vi "Test Formula.vi"() -> ()   [LabVIEW 2021]
uses:
  WHH Formula Data.ctl
panel:
  in  "alpha_Maki":dbl
  out "Array - Numeric":dbl[](array[numeric])
  out "XY Graph":cluster{dbl[], "Steps":dbl[]}(graph)
  in  "Number of steps":i32=20
  in  "End":dbl=0.99
  in  "Start":dbl=1e-05
  in  "t":dbl=0.5
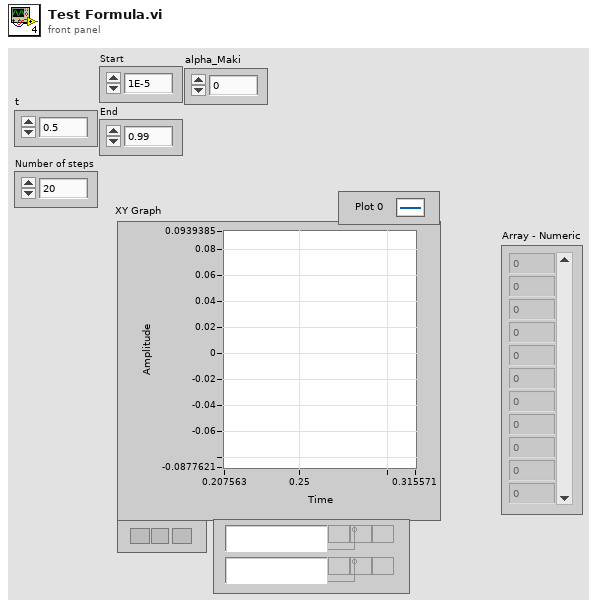
[diagram p1: front panel]
types:
  T1 = typedef "WHH Formula Data.ctl" = cluster{"t":dbl, "alpha_Maki":dbl, "lambda_SO":dbl}
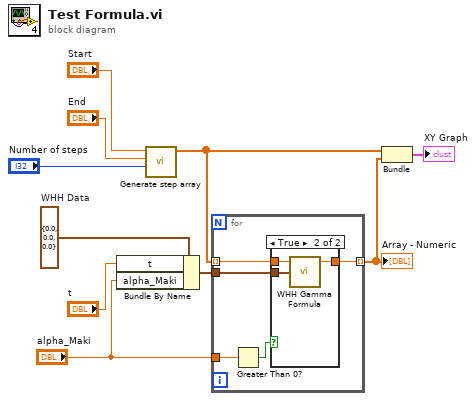
[diagram p0: block diagram]
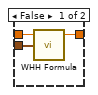
[diagram p2: hidden frame]
diagram:
  w10 = T1 {"t"=0.0, "alpha_Maki"=0.0, "lambda_SO"=0.0}  # WHH Data
  n1 = Bundle By Name(cluster=w10, "t"="t", "alpha_Maki"="alpha_Maki") -> (w9:T1)
  n2 = call "Generate step array.vi"("Number of steps"="Number of steps", "End"="End", "Start"="Start") -> ("Steps"=w3:dbl[])  [unwired: 8 in]
  n3 = for {
    tunnel: w9 -> [w15]
    tunnel: w3 -> [w14] mode=indexing
    tunnel: [w13] -> w4 mode=indexing
    tunnel: "alpha_Maki" -> [w11]
    n4 = Greater Than 0?(x=w11) -> (x > 0?=w12:bool)
    n5 = case shown="True" w12 {
      tunnel: w15 -> [w18 w20]
      tunnel: w14 -> [w17 w21]
      tunnel: [w16 w19] -> w13
      frame False {
        n6 = call "WHH Formula.vi"("data"=w18, "x"=w17) -> ("WHH(x)"=w16:dbl)  [unwired: 3 in]
      }
      frame True {
        n7 = call "WHH Gamma Formula.vi"("data"=w20, "x"=w21) -> ("WHH(x)"=w19:dbl)  [unwired: 3 in]
      }
    }
  }
  "Array - Numeric" <- w4
  n8 = Bundle("Steps"=w3, w4) -> (→"XY Graph":cluster{"Steps":dbl[], dbl[]})  [unwired: 1 in]
